vi "niRFUtil FTW Generate Synchronously Tuned Response.vi"(0 "Center Frequency (Hz)":dbl format="%^.6e", 1 "Bandwidth (Hz)":T3 format="%^.3e", 2 "df (Hz)":dbl format="%^.2e", 3 "Minimum Selectivity (dB)":dbl=70.0 format="%.2f", 4 "Poles (5)":i32=5) -> (5 "Filter Power Response":T1 {"y" min=0 max=127 format="%.2f"; "dx" format="%^.2e"; "x0" format="%^.2e"}, 6 "-ENBW (dB-Hz)":sgl format="%.2f")   [LabVIEW 2015, in "niRFUtil.lvlib"]
doc: "(c) Copyright 2006, National Instruments, Inc. This VI may not be duplicated, sold, or distributed without written consent from National Instruments."
uses:
  niRFUtil.lvlib
  Includes/niRFUtil INC RBW Filter Bandwidth.ctl
  Includes/niRFUtil INC Real Waveform.ctl
  Includes/niRFUtil INC Real Array.ctl
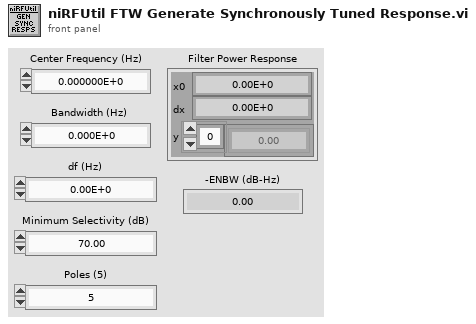
[diagram p1: front panel]
types:
  T1 = typedef "niRFUtil.lvlib/niRFUtil INC Real Waveform.ctl" = cluster{"x0":dbl, "dx":dbl, "y":T2}
  T2 = typedef "niRFUtil.lvlib/niRFUtil INC Real Array.ctl" = sgl[]
  T3 = typedef "niRFUtil.lvlib/niRFUtil INC RBW Filter Bandwidth.ctl" = dbl
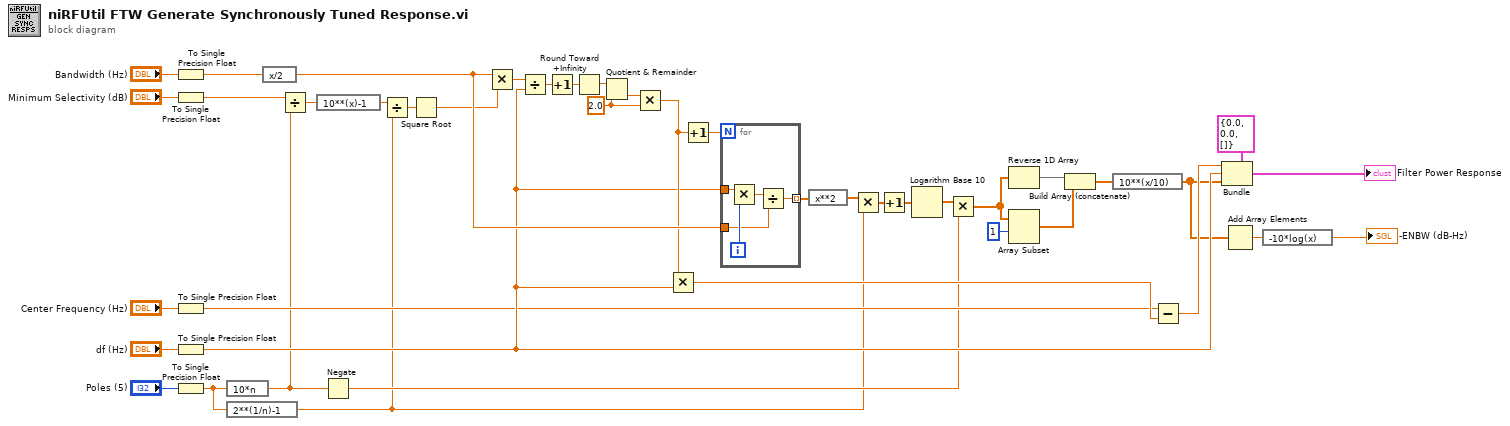
[diagram p0: block diagram]
diagram:
  w33 = sgl 2.0 ("y")
  n1 = To Single Precision Float(number="Bandwidth (Hz)") -> (single precision float=w19:sgl)
  n2 = To Single Precision Float(number="Minimum Selectivity (dB)") -> (single precision float=w14:sgl)
  n3 = To Single Precision Float(number="Center Frequency (Hz)") -> (single precision float=w22:sgl)
  n4 = To Single Precision Float(number="df (Hz)") -> (single precision float=w24:sgl)
  n5 = To Single Precision Float(number="Poles (5)") -> (single precision float=w13:sgl)
  n6 = expression code="10*n"(w13) -> (w9:sgl)
  n7 = expression code="2**(1/n)-1"(w13) -> (w2:sgl)
  n8 = expression code="x/2"(w19) -> (w37:sgl)
  n9 = Divide(x=w14, y=w9) -> (x/y=w12:sgl)
  n10 = expression code="10**(x)-1"(w12) -> (w11:sgl)
  n11 = Negate(x=w9) -> (-x=w7:sgl)
  n12 = Divide(x=w11, y=w2) -> (x/y=w10:sgl)
  n13 = Square Root(x=w10) -> (sqrt(x)=w3:sgl)
  n14 = Multiply(x=w37, y=w3) -> (x*y=w43:sgl)
  n15 = Divide(x=w43, y=w24) -> (x/y=w31:sgl)
  n16 = Increment(x=w31) -> (x+1=w32:sgl)
  n17 = Round Toward +Infinity(x=w32) -> (ceil(x): smallest int >= x=w35:sgl)
  n18 = Quotient & Remainder(x=w35, y=w33) -> (floor(x/y)=w34:sgl)  [unwired: 1 out]
  n19 = Multiply(x=w34, y=w33) -> (x*y=w30:sgl)
  n20 = Multiply(x=w30, y=w24) -> (x*y=w36:sgl)
  n21 = Increment(x=w30) -> (x+1=w38:sgl)
  n22 = for {
    N: w38 -> [_]
    tunnel: w24 -> [w48]
    tunnel: w37 -> [w45]
    tunnel: [w44] -> w42 mode=indexing
    i -> [w47]
    n23 = Multiply(x=w48, y=w47) -> (x*y=w46:sgl)
    n24 = Divide(x=w46, y=w45) -> (x/y=w44:sgl)
  }
  n25 = expression code="x**2"(w42) -> (w5:sgl[])
  n26 = Multiply(x=w5, y=w2) -> (x*y=w4:sgl[])
  n27 = Increment(x=w4) -> (x+1=w1:sgl[])
  n28 = Logarithm Base 10(1:w1) -> (0:w6:sgl[])
  n29 = Multiply(x=w6, y=w7) -> (x*y=w8:sgl[])
  n30 = Reverse 1D Array(array=w8) -> (reversed array=w41:sgl[])
  n31 = Array Subset(array=w8, index=1) -> (w40:sgl[])  [unwired: 1 in]
  n32 = Build Array (concatenate)(w41, w40) -> (w29:sgl[])
  n33 = expression code="10**(x/10)"(w29) -> (w17:sgl[])
  n34 = Subtract(x=w22, y=w36) -> (x-y=w28:sgl)
  n35 = Bundle(cluster=T1 {"x0"=0.0, "dx"=0.0, "y"=[]} ("Filter"), "x0"=w28, "dx"=w24, "y"=w17) -> (→"Filter Power Response":T1)
  n36 = Add Array Elements(numeric array=w17) -> (sum=w18:sgl)
  n37 = expression code="-10*log(x)"(w18) -> (→"-ENBW (dB-Hz)":sgl)
